vi "Build Tree.vi"(8 "error in":errorcluster, 11 "Project in":refnum<class "Project.lvclass">) -> (0 "error out":errorcluster, 2 "Tree Map Out":T1, 3 "Project Out":refnum<class "Project.lvclass">)   [LabVIEW 2019, in "Panther Dashboard.lvlib" / "Project.lvclass"]
uses:
  Project.lvclass
  C:/GitClones/PantherDashboard/src/LabVIEW/Panther Dashboard/Class/LabVIEWItem/LabVIEWItem.lvclass
  <vilib>/National Instruments/Tree Map/Tree Map Data.ctl
  Panther Dashboard/Map Attribute--enum.ctl
  Project.lvclass/Project.ctl
  LabVIEWItem/LabVIEWItem.lvclass/LabVIEWItem.ctl
  Library/Library.lvclass/Library.ctl
  LabVIEWItem/Read Item Name.vi
  LabVIEWItem/Read Item Path.vi
  LabVIEWItem/Write Item Tag.vi
  Library/Read VIs MAP.vi
  Library/Read Type.vi
  Library/Read Dependency.vi
  Library/Write VIs MAP.vi
  Read Libraries.vi
  Read Target Name.vi
  Write Libraries.vi
  Library/Library.lvclass
  VI/VI.lvclass
  <vilib>/National Instruments/Tree Map/Tree Map.lvlib
  Panther Dashboard/Panther Dashboard.lvlib
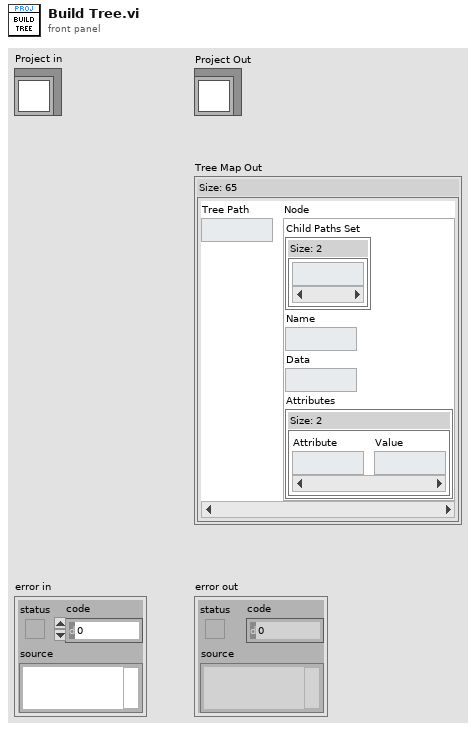
[diagram p1: front panel]
types:
  T1 = typedef "Tree Map.lvlib/Tree Map Data.ctl" = map{string, cluster{"Child Paths Set":set{string}, "Name":string, "Data":string, "Attributes":map{string, string}}}
  T2 = typedef "Panther Dashboard.lvlib/Map Attribute--enum.ctl" = enum16{"Path", "ModuleType", "Module Description", "Dependency?", "Target"}
  T3 = typedef "Panther Dashboard.lvlib/LabVIEWItem.lvclass/VI Type--enum.ctl" = enum16{"Requests", "Broadcasts", "Request and Wait for Reply", "Round Trip", "Public API VIs", "» Constant VIs", "» Error VIs", "Module", "Project"}
  T4 = typedef "Panther Dashboard.lvlib/Module type--enum.ctl" = enum16{"Singleton", "Cloneable"}
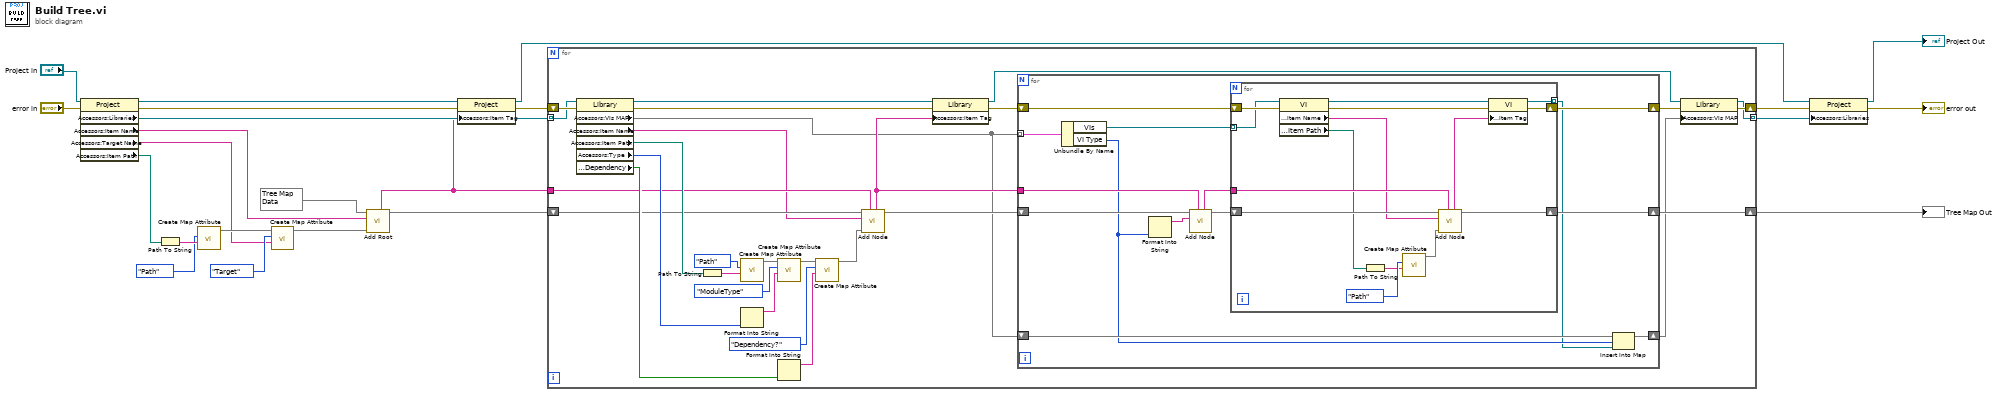
[diagram p0: block diagram]
diagram:
  n1 = property class="Project"(reference="Project in", error in="error in") -> (reference out=w5:refnum<class "Project.lvclass">, error out=w22:errorcluster, "Accessors:Libraries"=w10:refnum<class "Library.lvclass">[], "Accessors:Item Name"=w11:string, "Accessors:Target Name"=w7:string, "Accessors:Item Path"=w8:path)
  n2 = Path To String(path=w8) -> (string=w17:string)
  n3 = call "Create Map Attribute.vi"("Attribute"=w17, "Map Attribute"=Map_Attribute--enum."Path") -> ("Root Attributes"=w16:map{string, string})  [unwired: 9 in]
  n4 = call "Create Map Attribute.vi"("Attribute"=w7, "Map Attribute"=Map_Attribute--enum."Target", "Root Attributes In"=w16) -> ("Root Attributes"=w15:map{string, string})  [unwired: 8 in]
  n5 = call <vilib>:"Add Root.vi"("Root Attributes"=w15, "New Root Name"=w11, "Tree Map In"=T1 {} ("Tree Map out")) -> ("Tree Map Out"=w9:T1, "Root Path"=w4:string)  [unwired: 7 in]
  n6 = property class="Project"(reference=w5, error in=w22, "Accessors:Item Tag"=w4) -> (reference out=w3:refnum<class "Project.lvclass">, error out=w20:errorcluster)
  n7 = for {
    shift-right: [w48] -> w21
    shift-left: w20 -> [w52]
    tunnel: w10 -> [w47] mode=indexing
    shift-right: [w30] -> w6
    shift-left: w9 -> [w35]
    tunnel: w4 -> [w33]
    tunnel: [w27] -> w1 mode=indexing
    n8 = property class="Library"(reference=w47, error in=w52) -> (reference out=w29:refnum<class "Library.lvclass">, error out=w51:errorcluster, "Accessors:VIs MAP"=w26:map{T3, refnum<class "VI.lvclass">[]}, "Accessors:Item Name"=w32:string, "Accessors:Item Path"=w45:path, "Accessors:Type"=w41:T4, "Accessors:Dependency"=w37:bool)
    n9 = Path To String(path=w45) -> (string=w42:string)
    n10 = call "Create Map Attribute.vi"("Attribute"=w42, "Map Attribute"=Map_Attribute--enum."Path") -> ("Root Attributes"=w44:map{string, string})  [unwired: 9 in]
    n11 = Format Into String(w41) -> (resulting string=w38:string)  [unwired: 3 in, 1 out]
    n12 = call "Create Map Attribute.vi"("Attribute"=w38, "Map Attribute"=Map_Attribute--enum."ModuleType", "Root Attributes In"=w44) -> ("Root Attributes"=w40:map{string, string})  [unwired: 8 in]
    n13 = Format Into String(w37) -> (resulting string=w36:string)  [unwired: 3 in, 1 out]
    n14 = call "Create Map Attribute.vi"("Attribute"=w36, "Map Attribute"=Map_Attribute--enum."Dependency?", "Root Attributes In"=w40) -> ("Root Attributes"=w34:map{string, string})  [unwired: 8 in]
    n15 = call <vilib>:"Add Node.vi"("Parent Path"=w33, "Attributes"=w34, "New Node Name"=w32, "Tree Map In"=w35) -> ("Tree Map Out"=w31:T1, "New Node Path"=w28:string)  [unwired: 5 in, 1 out]
    n16 = property class="Library"(reference=w29, error in=w51, "Accessors:Item Tag"=w28) -> (reference out=w25:refnum<class "Library.lvclass">, error out=w49:errorcluster)
    n17 = for {
      shift-right: [w61] -> w30
      shift-left: w31 -> [w64]
      shift-right: [w65] -> w50
      shift-left: w49 -> [w66]
      tunnel: w28 -> [w62]
      tunnel: w26 -> [w58] mode=indexing
      shift-right: [w56] -> w24
      shift-left: w26 -> [w55]
      n18 = Unbundle By Name(w58) -> ("VIs"=w57:refnum<class "VI.lvclass">[], "VI Type"=w54:T3)
      n19 = Format Into String(w54) -> (resulting string=w59:string)  [unwired: 3 in, 1 out]
      n20 = call <vilib>:"Add Node.vi"("Parent Path"=w62, "New Node Name"=w59, "Tree Map In"=w64) -> ("Tree Map Out"=w63:T1, "New Node Path"=w60:string)  [unwired: 6 in, 1 out]
      n21 = for {
        tunnel: w60 -> [w76]
        shift-right: [w79] -> w65
        shift-left: w66 -> [w81]
        shift-right: [w77] -> w61
        shift-left: w63 -> [w78]
        tunnel: w57 -> [w70] mode=indexing
        tunnel: [w67] -> w53 mode=indexing
        n22 = property class="VI"(reference=w70, error in=w81) -> (reference out=w69:refnum<class "VI.lvclass">, error out=w80:errorcluster, "Accessors:Item Name"=w72:string, "Accessors:Item Path"=w71:path)
        n23 = Path To String(path=w71) -> (string=w73:string)
        n24 = call "Create Map Attribute.vi"("Attribute"=w73, "Map Attribute"=Map_Attribute--enum."Path") -> ("Root Attributes"=w74:map{string, string})  [unwired: 9 in]
        n25 = call <vilib>:"Add Node.vi"("Parent Path"=w76, "Attributes"=w74, "New Node Name"=w72, "Tree Map In"=w78) -> ("Tree Map Out"=w77:T1, "New Node Path"=w68:string)  [unwired: 5 in, 1 out]
        n26 = property class="VI"(reference=w69, error in=w80, "Accessors:Item Tag"=w68) -> (reference out=w67:refnum<class "VI.lvclass">, error out=w79:errorcluster)
      }
      n27 = Insert Into Map(map in=w55, key=w54, value=w53) -> (map out=w56:map{T3, refnum<class "VI.lvclass">[]})  [unwired: 2 out]
    }
    n28 = property class="Library"(reference=w25, error in=w50, "Accessors:VIs MAP"=w24) -> (reference out=w27:refnum<class "Library.lvclass">, error out=w48:errorcluster)
  }
  "Tree Map Out" <- w6
  n29 = property class="Project"(reference=w3, error in=w21, "Accessors:Libraries"=w1) -> (reference out=→"Project Out":refnum<class "Project.lvclass">, error out=→"error out":errorcluster)
